vi "Add Cashier.vi"(8 "error in (no error)":errorcluster, 10 "Name":string, 11 "Coffee Shop in":refnum<class "Coffee Shop.lvclass">) -> (0 "error out":errorcluster, 3 "Coffee Shop out":refnum<class "Coffee Shop.lvclass">)   [LabVIEW 2020, in "Coffee Shop.lvclass"]
uses:
  Coffee Shop.lvclass
  C:/Program Files (x86)/National Instruments/LabVIEW 2020/vi.lib/Asteme/Triarc Framework/Process/Process.lvclass
  Cashier/Cashier.lvclass
  <vilib>/Asteme/Triarc Framework/Process/Process.lvclass/Process.ctl
  <vilib>/Asteme/Triarc Framework/Process/Public/Lifecycle/Get Lifecycle State.vi
  <vilib>/Utility/error.llb/Clear Errors.vi
  <vilib>/Utility/error.llb/Error Cluster From Error Code.vi
  <vilib>/Asteme/Triarc Framework/Process/Process.lvclass
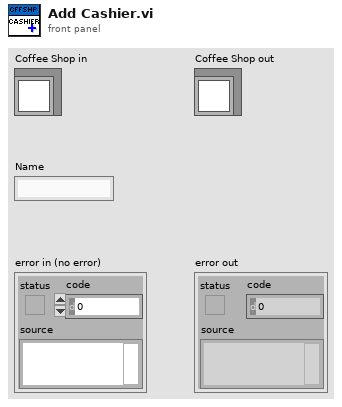
[diagram p1: front panel]
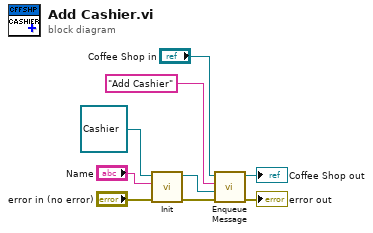
[diagram p0: block diagram]
diagram:
  n1 = call-dynamic "Init.vi"("error in (no error)"="error in (no error)", "Name"="Name", "View In"=refnum<class "Cashier.lvclass"> refnum ("Cashier.lvclass")) -> ("error out"=w2:errorcluster, "View Out"=w1:refnum<class "Cashier.lvclass">)  [unwired: 7 in]
  n2 = call <vilib>:"Enqueue Message.vi"("error in (no error)"=w2, "Message Data"=w1, "Message"="Add Cashier", "Process In"="Coffee Shop in") -> ("error out"=→"error out":errorcluster, "Process Out"=→"Coffee Shop out":refnum<class "Coffee Shop.lvclass">)  [unwired: 6 in]
